vi "GetParam.vi"(8 "error in (no error)":errorcluster caption="entrée d'erreur (pas d'erreur)", 11 "GaussianRandomProjection.lvclass":refnum<class "GaussianRandomProjection.lvclass">) -> (0 "error out":errorcluster caption="sortie d'erreur", 2 "GaussianRandomProjection":T1={"n_components"="auto", "eps"=0.1, "random_state"=-1} {"random_state" min=-1; "eps" min=0.0}, 3 "GaussianRandomProjection.lvclass":refnum<class "GaussianRandomProjection.lvclass">)   [LabVIEW 2020, in "GaussianRandomProjection.lvclass"]
doc: "Get Parameters"
uses:
  GaussianRandomProjection.lvclass
  GaussianRandomProjection.lvclass/GaussianRandomProjection.ctl
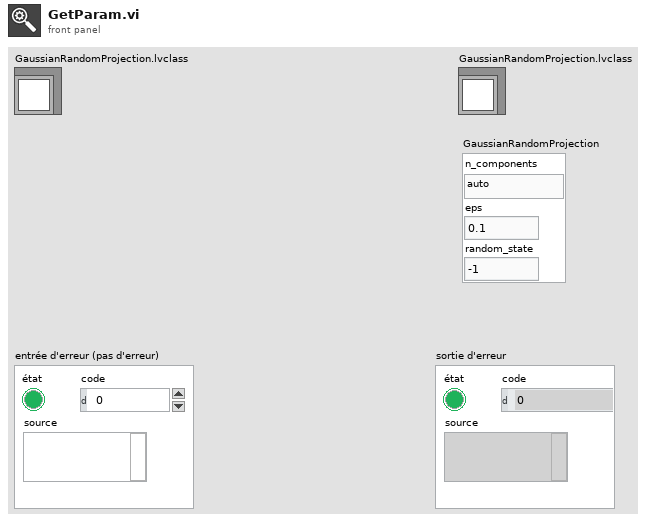
[diagram p1: front panel]
types:
  T1 = cluster{"n_components":string, "eps":dbl, "random_state":i32}
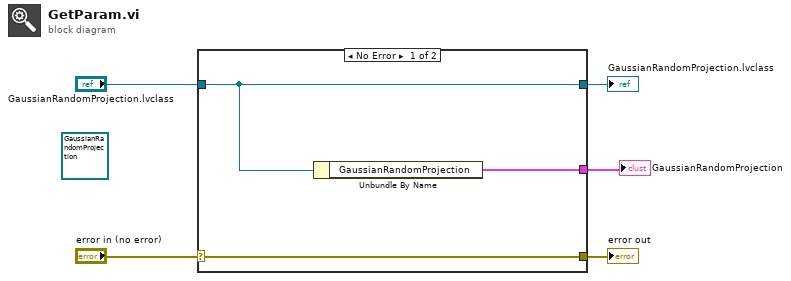
[diagram p0: block diagram]
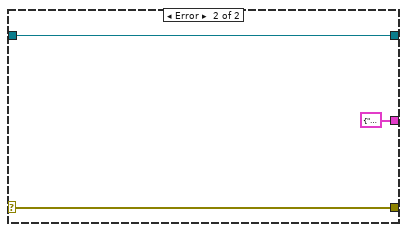
[diagram p2: hidden frame]
diagram:
  (unwired) refnum<class "GaussianRandomProjection.lvclass"> refnum ("GaussianRandomProjection.lvclass")
  n1 = case shown="No Error" "error in (no error)" {
    selector: "error in (no error)" -> [w8 w10]
    tunnel: [w8 w10] -> w4
    tunnel: [w7 w11] -> w2
    tunnel: "GaussianRandomProjection.lvclass" -> [w7 w11]
    tunnel: [w6 T1 {"n_components"="", "eps"=0.0, "random_state"=0} ("GaussianRandomProjection")] -> w1
    frame No Error {
      n2 = Unbundle By Name(w7) -> ("GaussianRandomProjection"=w6:T1)
    }
    frame Error {
    }
  }
  "error out" <- w4
  "GaussianRandomProjection.lvclass" <- w2
  "GaussianRandomProjection" <- w1
